vi "insert 2 serials in the begining.vi"(8 "error in (no error)":errorcluster, 10 "Seials array":string[](array[string]), 11 "Domino Laser module Class in":refnum<class "Domino Laser module Class.lvclass">) -> (0 "error out":errorcluster, 2 "array w/ subset deleted":string[](array[string]), 3 "Domino Laser module Class out":refnum<class "Domino Laser module Class.lvclass">)   [LabVIEW 2015, in "Domino LM.lvlib" / "Domino Laser module Class.lvclass"]
uses:
  CTRLS/Domino Laser module Class.lvclass
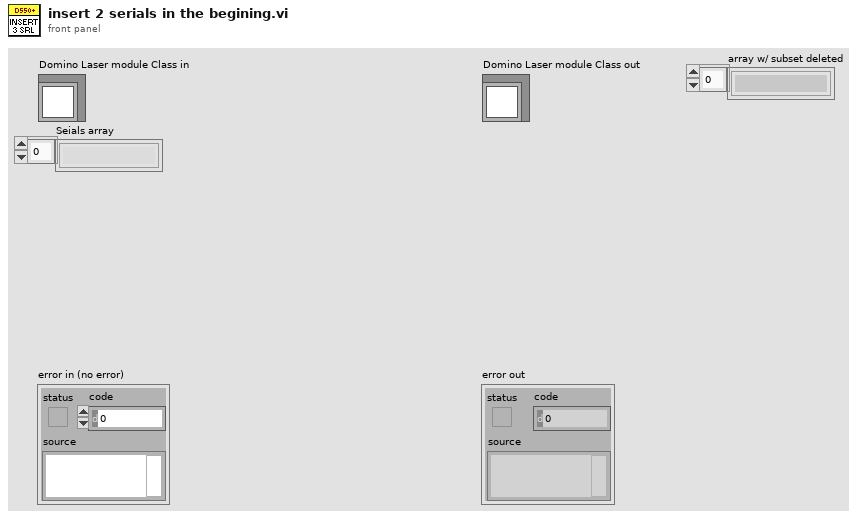
[diagram p1: front panel]
types:
  T1 = enum16{"Init SRL Buffer", "Insert SRL in Buffer", "Insert SRL Status", "Remove SRL from Buffer"}
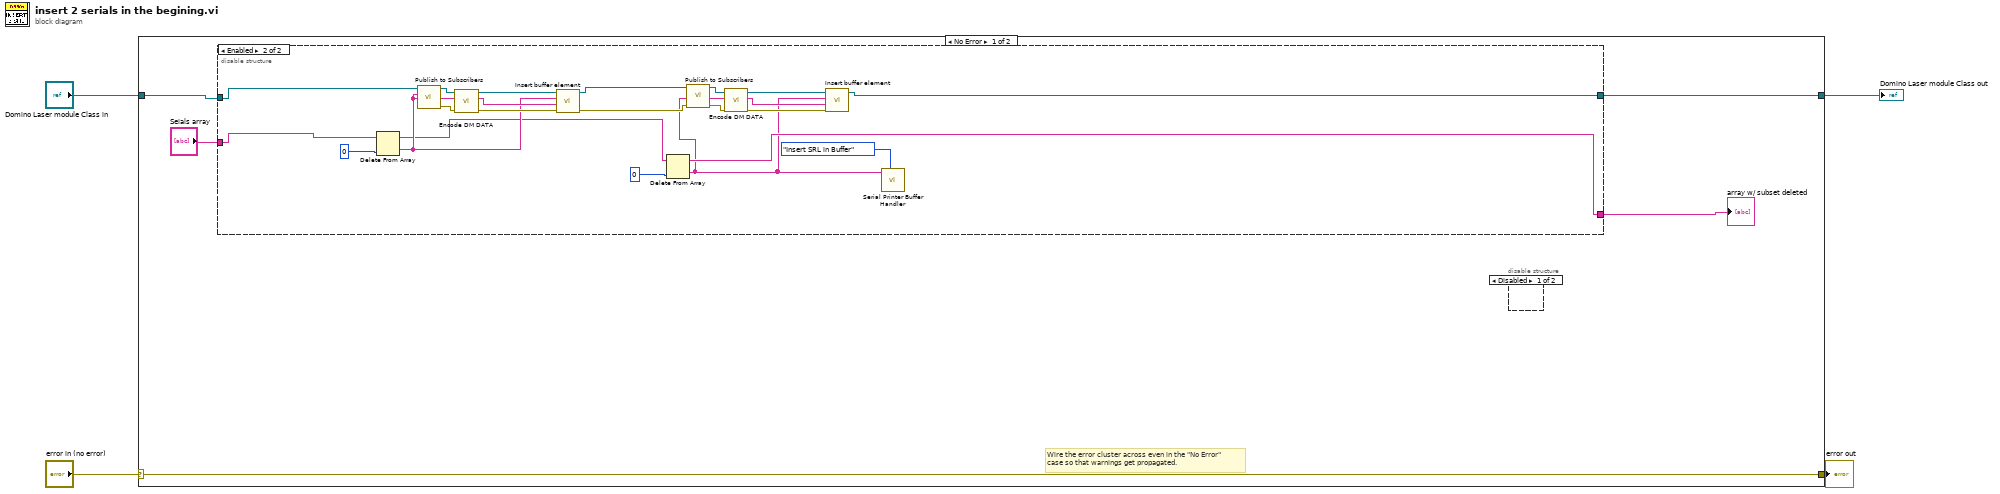
[diagram p0: block diagram]
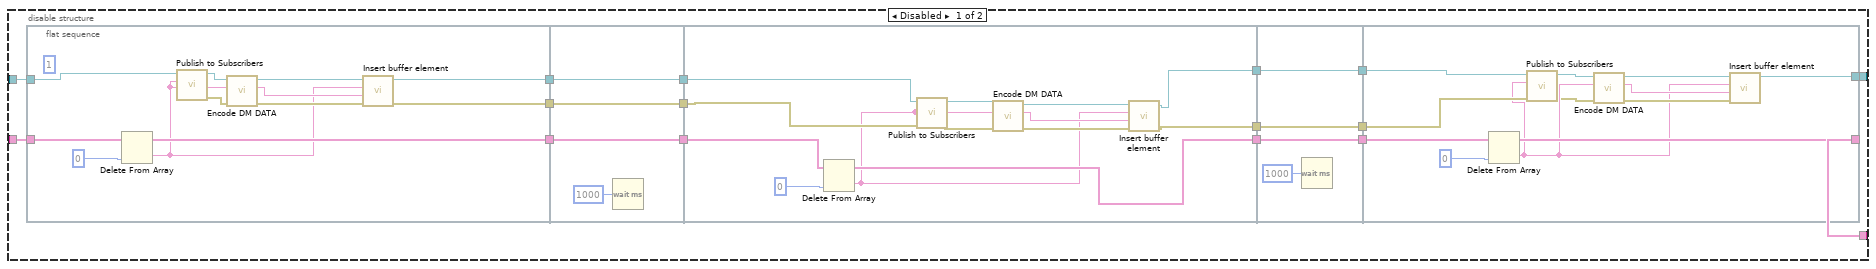
[diagram p2: hidden frame]
diagram:
  n1 = case shown="No Error" "error in (no error)" {
    selector: "error in (no error)" -> [w9 w93]
    tunnel: [w9 w93] -> w3
    tunnel: [w6 w92] -> w1
    tunnel: "Domino Laser module Class in" -> [w8 w92]
    frame No Error {
      # "Wire the error cluster across even in the \"No Error\"\ncase so that warnings get propagated."
      n2 = disable-structure shown="Enabled" {
        disable-tunnel: w8 -> [w13 w91]
        disable-tunnel: "Seials array" -> [w12 w90]
        disable-tunnel: [w11 w77] -> w6
        disable-tunnel: [w10 w78] -> w5
        frame Disabled {
          n3 = flat-sequence {
            tunnel: w13 -> [w31]
            tunnel: w12 -> [w37]
            tunnel: [w36] -> w25
            tunnel: [w27] -> w24
            tunnel: [w26] -> w23
            tunnel: w25 -> [w41]
            tunnel: [w41] -> w22
            tunnel: [w40] -> w21
            tunnel: [w39] -> w20
            tunnel: w24 -> [w40]
            tunnel: w23 -> [w39]
            tunnel: w22 -> [w50]
            tunnel: w21 -> [w46]
            tunnel: w20 -> [w43]
            tunnel: [w49] -> w19
            tunnel: [w48] -> w18
            tunnel: [w47] -> w17
            tunnel: w19 -> [w58]
            tunnel: [w58] -> w16
            tunnel: [w57] -> w15
            tunnel: w18 -> [w57]
            tunnel: [w55] -> w14
            tunnel: w17 -> [w55]
            tunnel: [w65] -> w10
            tunnel: w16 -> [w65]
            tunnel: w15 -> [w63]
            tunnel: [w64] -> w11
            tunnel: w14 -> [w62]
            frame #0 {
              (unwired) 1
              n4 = Delete From Array "Delete From Array"(array=w37, index=0) -> (deleted portion=w28:string, array with subset deleted=w36:string[])  [unwired: 1 in]
              n5 = call "Publish to Subscribers.vi"("Message Data"=w28, "Domino Laser module Class in"=w31) -> ("error out"=w29:errorcluster, "Domino Laser module Class out"=w30:refnum<class "Domino Laser module Class.lvclass">)  [unwired: 8 in]
              n6 = call "Encode DM DATA.vi"("error in (no error)"=w29, "serial"=w28, "Domino Laser module Class in"=w30) -> ("error out"=w32:errorcluster, "DM"=w34:string, "Domino Laser module Class out"=w35:refnum<class "Domino Laser module Class.lvclass">)  [unwired: 6 in]
              n7 = call "Insert buffer element.vi"("error in (no error)"=w32, "DM"=w34, "Serial"=w28, "Domino Laser module Class in"=w35) -> ("error out"=w26:errorcluster, "Domino Laser module Class out"=w27:refnum<class "Domino Laser module Class.lvclass">)  [unwired: 5 in, 1 out]
            }
            frame #1 {
              n8 = Wait (ms)(milliseconds to wait=u32 1000) -> ()  [unwired: 1 out]
            }
            frame #2 {
              n9 = Delete From Array "Delete From Array"(array=w50, index=0) -> (deleted portion=w42:string, array with subset deleted=w49:string[])  [unwired: 1 in]
              n10 = call "Publish to Subscribers.vi"("error in (no error)"=w43, "Message Data"=w42, "Domino Laser module Class in"=w46) -> ("error out"=w44:errorcluster, "Domino Laser module Class out"=w45:refnum<class "Domino Laser module Class.lvclass">)  [unwired: 7 in]
              n11 = call "Encode DM DATA.vi"("error in (no error)"=w44, "serial"=w42, "Domino Laser module Class in"=w45) -> ("error out"=w54:errorcluster, "DM"=w52:string, "Domino Laser module Class out"=w53:refnum<class "Domino Laser module Class.lvclass">)  [unwired: 6 in]
              n12 = call "Insert buffer element.vi"("error in (no error)"=w54, "DM"=w52, "Serial"=w42, "Domino Laser module Class in"=w53) -> ("error out"=w47:errorcluster, "Domino Laser module Class out"=w48:refnum<class "Domino Laser module Class.lvclass">)  [unwired: 5 in, 1 out]
            }
            frame #3 {
              n13 = Wait (ms)(milliseconds to wait=u32 1000) -> ()  [unwired: 1 out]
            }
            frame #4 {
              n14 = Delete From Array "Delete From Array"(array=w65, index=0) -> (deleted portion=w61:string)  [unwired: 1 in, 1 out]
              n15 = call "Publish to Subscribers.vi"("error in (no error)"=w62, "Message Data"=w61, "Domino Laser module Class in"=w63) -> ("error out"=w59:errorcluster, "Domino Laser module Class out"=w60:refnum<class "Domino Laser module Class.lvclass">)  [unwired: 7 in]
              n16 = call "Encode DM DATA.vi"("error in (no error)"=w59, "serial"=w61, "Domino Laser module Class in"=w60) -> ("error out"=w66:errorcluster, "DM"=w68:string, "Domino Laser module Class out"=w67:refnum<class "Domino Laser module Class.lvclass">)  [unwired: 6 in]
              n17 = call "Insert buffer element.vi"("error in (no error)"=w66, "DM"=w68, "Serial"=w61, "Domino Laser module Class in"=w67) -> ("Domino Laser module Class out"=w64:refnum<class "Domino Laser module Class.lvclass">)  [unwired: 5 in, 2 out]
            }
          }
        }
        frame Enabled {
          n18 = Delete From Array "Delete From Array"(array=w90, index=0) -> (deleted portion=w83:string, array with subset deleted=w79:string[])  [unwired: 1 in]
          n19 = call "Publish to Subscribers.vi"("Message Data"=w83, "Domino Laser module Class in"=w91) -> ("error out"=w84:errorcluster, "Domino Laser module Class out"=w85:refnum<class "Domino Laser module Class.lvclass">)  [unwired: 8 in]
          n20 = call "Encode DM DATA.vi"("error in (no error)"=w84, "serial"=w83, "Domino Laser module Class in"=w85) -> ("error out"=w86:errorcluster, "DM"=w88:string, "Domino Laser module Class out"=w89:refnum<class "Domino Laser module Class.lvclass">)  [unwired: 6 in]
          n21 = call "Insert buffer element.vi"("error in (no error)"=w86, "DM"=w88, "Serial"=w83, "Domino Laser module Class in"=w89) -> ("error out"=w81:errorcluster, "Domino Laser module Class out"=w82:refnum<class "Domino Laser module Class.lvclass">)  [unwired: 5 in, 1 out]
          n22 = Delete From Array "Delete From Array"(array=w79, index=0) -> (deleted portion=w70:string, array with subset deleted=w78:string[])  [unwired: 1 in]
          n23 = call "Publish to Subscribers.vi"("error in (no error)"=w81, "Domino Laser module Class in"=w82) -> ("error out"=w75:errorcluster, "Domino Laser module Class out"=w74:refnum<class "Domino Laser module Class.lvclass">)  [unwired: 8 in]
          n24 = call "Encode DM DATA.vi"("error in (no error)"=w75, "serial"=w70, "Domino Laser module Class in"=w74) -> ("error out"=w73:errorcluster, "DM"=w72:string, "Domino Laser module Class out"=w71:refnum<class "Domino Laser module Class.lvclass">)  [unwired: 6 in]
          n25 = call "Insert buffer element.vi"("error in (no error)"=w73, "DM"=w72, "Serial"=w70, "Domino Laser module Class in"=w71) -> ("Domino Laser module Class out"=w77:refnum<class "Domino Laser module Class.lvclass">)  [unwired: 5 in, 2 out]
          n26 = call "Serial Printer Buffer Handler.vi"("Serials buffer operations"=T1."Insert SRL in Buffer", "Serial"=w70) -> ()  [unwired: 8 in, 2 out]
        }
      }
      "array w/ subset deleted" <- w5
      n27 = disable-structure shown="Disabled" {
        frame Disabled {
        }
        frame Enabled {
        }
      }
    }
    frame Error {
    }
  }
  "error out" <- w3
  "Domino Laser module Class out" <- w1
